vi "Convert Raw Bus Monitor Log.vi"(7 "48-bit Timetag?":bool, 8 "error in (no error)":errorcluster, 11 "Raw Bus Monitor Log":u16[](array[numeric])) -> (0 "error out":errorcluster, 3 "Formatted Bus Monitor Log":string[][](array[string]))   [LabVIEW 2016, in "BCI-1553 API.lvlib" / "1553 Component.lvclass"]
doc: "Converts a raw bus monitor log to a human-readable format. The first row is a header."
uses:
  1553 Component.lvclass
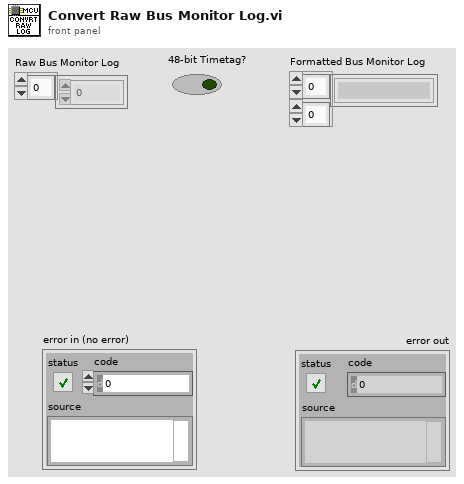
[diagram p1: front panel]
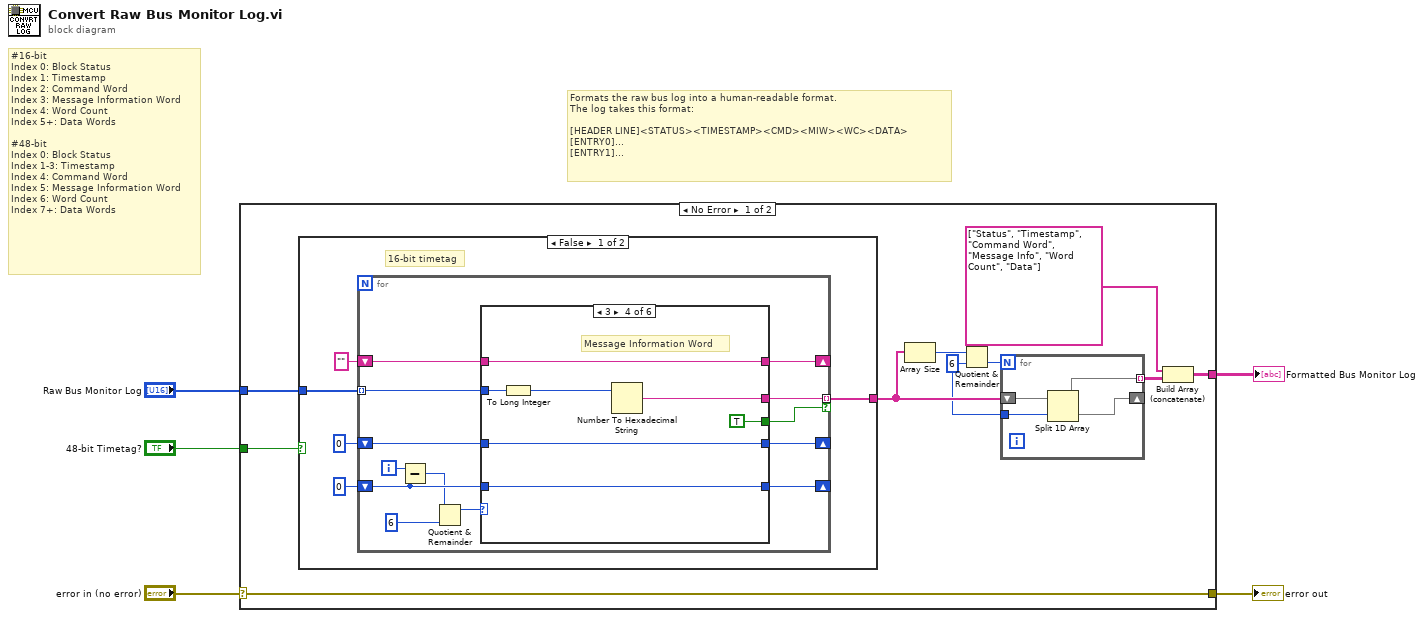
[diagram p0: block diagram]
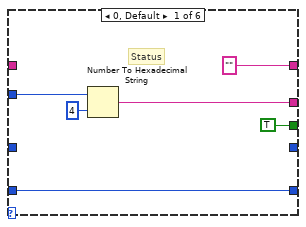
[diagram p2: hidden frame]
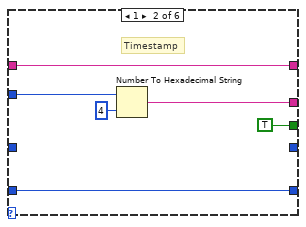
[diagram p3: hidden frame]
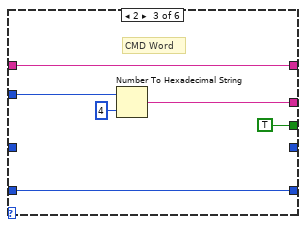
[diagram p4: hidden frame]
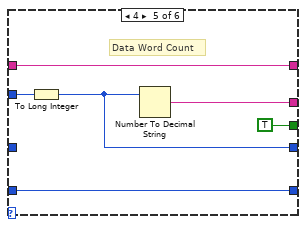
[diagram p5: hidden frame]
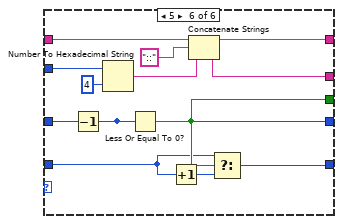
[diagram p6: hidden frame]
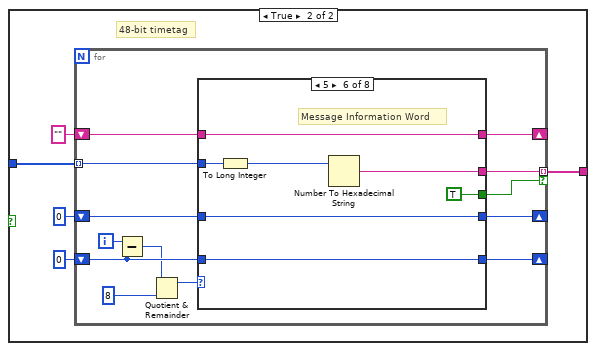
[diagram p7: hidden frame]
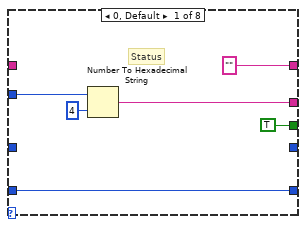
[diagram p8: hidden frame]
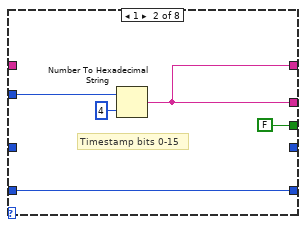
[diagram p9: hidden frame]
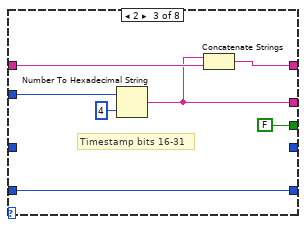
[diagram p10: hidden frame]
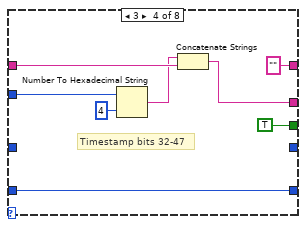
[diagram p11: hidden frame]
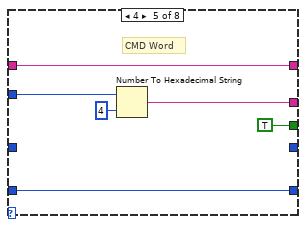
[diagram p12: hidden frame]
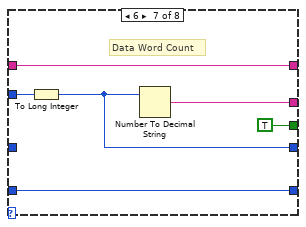
[diagram p13: hidden frame]
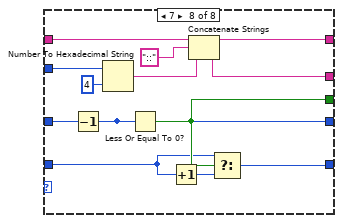
[diagram p14: hidden frame]
diagram:
  # "#16-bit\nIndex 0: Block Status\nIndex 1: Timestamp\nIndex 2: Command Word\nIndex 3: Message Information Word\nIndex 4: Word Count\nIndex 5+: Data Words\n\n#48-bit\nIndex 0: Block Status\nIndex 1-3: Timestamp\nIndex 4: Command Word\nIndex 5: Message Information Word\nIndex 6: Word Count\nIndex 7+: Data Words"
  # "Formats the raw bus log into a human-readable format.\nThe log takes this format:\n\n[HEADER LINE]<STATUS><TIMESTAMP><CMD><MIW><WC><DATA>\n[ENTRY0]...\n[ENTRY1]..."
  n1 = case shown="No Error" "error in (no error)" {
    selector: "error in (no error)" -> [w15 w156]
    tunnel: [w15 w156] -> w2
    tunnel: "Raw Bus Monitor Log" -> [w14 _]
    tunnel: [w8 _] -> w3
    tunnel: "48-bit Timetag?" -> [w6 _]
    frame No Error {
      w10 = 6 ("y")
      n2 = case shown="False" w6 {
        tunnel: w14 -> [w20 w78]
        tunnel: [w16 w77] -> w13
        frame False {
          # "16-bit timetag"
          n3 = for {
            tunnel: w20 -> [w27] mode=indexing
            shift-right: [w31] -> _
            shift-left: 0 ("y") -> [w29]
            tunnel: [w26] -> w16 mode=indexing if=w23
            shift-right: [w25] -> _
            shift-left: "" -> [w24]
            shift-right: [w22] -> _
            shift-left: 0 -> [w21]
            i -> [w30]
            n4 = Subtract(x=w30, y=w29) -> (x-y=w28:i32)
            n5 = Quotient & Remainder(x=w28, y=6) -> (x-y*floor(x/y)=w32:i32)  [unwired: 1 out]
            n6 = case shown="3" w32 {
              tunnel: w29 -> [w39 w45 w51 w54 w60 w70]
              tunnel: [w39 w45 w51 w54 w60 w68] -> w31
              tunnel: w27 -> [w38 w42 w48 w56 w62 w76]
              tunnel: [w36 w41 w47 w55 w61 w72] -> w26
              tunnel: ["" w44 w50 w58 w64 w72] -> w25
              tunnel: w24 -> [_ w44 w50 w58 w64 w66]
              tunnel: [TRUE TRUE TRUE TRUE TRUE w71] -> w23
              tunnel: [_ _ _ w52 w59 w67] -> w22
              tunnel: w21 -> [_ _ _ w52 _ w74]
              frame 0, Default {
                # "Status"
                n7 = Number To Hexadecimal String(1:i16 4 ("width (-)"), 2:w38) -> (0:w36:string)
              }
              frame 1 {
                # "Timestamp"
                n8 = Number To Hexadecimal String(1:i16 4 ("width (-)"), 2:w42) -> (0:w41:string)
              }
              frame 2 {
                # "CMD Word"
                n9 = Number To Hexadecimal String(1:i16 4 ("width (-)"), 2:w48) -> (0:w47:string)
              }
              frame 3 {
                # "Message Information Word"
                n10 = To Long Integer(number=w56) -> (32bit integer=w53:i32)
                n11 = Number To Hexadecimal String(2:w53) -> (0:w55:string)  [unwired: 1 in]
              }
              frame 4 {
                # "Data Word Count"
                n12 = To Long Integer(number=w62) -> (32bit integer=w59:i32)
                n13 = Number To Decimal String(number=w59) -> (decimal integer string=w61:string)  [unwired: 1 in]
              }
              frame 5 {
                n14 = Decrement(x=w74) -> (x-1=w67:i32)
                n15 = Number To Hexadecimal String(1:i16 4 ("width (-)"), 2:w76) -> (0:w65:string)
                n16 = Less Or Equal To 0?(x=w67) -> (x <= 0?=w71:bool)
                n17 = Increment(x=w70) -> (x+1=w69:i32)
                n18 = Concatenate Strings(w66, "::" ("string"), w65) -> (w72:string)
                n19 = Select(t=w70, s=w71, f=w69) -> (s? t:f=w68:i32)
              }
            }
          }
        }
        frame True {
          # "48-bit timetag"
          n20 = for {
            tunnel: w78 -> [w88] mode=indexing
            shift-right: [w92] -> _
            shift-left: 0 ("y") -> [w90]
            tunnel: [w87] -> w77 mode=indexing if=w84
            shift-right: [w86] -> _
            shift-left: "" -> [w85]
            shift-right: [w83] -> _
            shift-left: 0 -> [w82]
            i -> [w91]
            n21 = Subtract(x=w91, y=w90) -> (x-y=w89:i32)
            n22 = Quotient & Remainder(x=w89, y=8) -> (x-y*floor(x/y)=w93:i32)  [unwired: 1 out]
            n23 = case shown="5" w93 {
              tunnel: w90 -> [w100 w105 w112 w120 w126 w129 w135 w145]
              tunnel: [w100 w105 w112 w120 w126 w129 w135 w143] -> w92
              tunnel: w88 -> [w99 w103 w110 w118 w123 w131 w137 w151]
              tunnel: [w97 w101 w107 w113 w122 w130 w136 w147] -> w87
              tunnel: ["" w101 w106 "" w125 w133 w139 w147] -> w86
              tunnel: w85 -> [_ _ w108 w115 w125 w133 w139 w141]
              tunnel: [TRUE FALSE FALSE TRUE TRUE TRUE TRUE w146] -> w84
              tunnel: [_ _ _ _ _ w127 w134 w142] -> w83
              tunnel: w82 -> [_ _ _ _ _ w127 _ w149]
              frame 0, Default {
                # "Status"
                n24 = Number To Hexadecimal String(1:i16 4 ("width (-)"), 2:w99) -> (0:w97:string)
              }
              frame 1 {
                # "Timestamp bits 0-15"
                n25 = Number To Hexadecimal String(1:i16 4 ("width (-)"), 2:w103) -> (0:w101:string)
              }
              frame 2 {
                # "Timestamp bits 16-31"
                n26 = Number To Hexadecimal String(1:i16 4 ("width (-)"), 2:w110) -> (0:w107:string)
                n27 = Concatenate Strings(w107, w108) -> (w106:string)
              }
              frame 3 {
                # "Timestamp bits 32-47"
                n28 = Number To Hexadecimal String(1:i16 4 ("width (-)"), 2:w118) -> (0:w114:string)
                n29 = Concatenate Strings(w114, w115) -> (w113:string)
              }
              frame 4 {
                # "CMD Word"
                n30 = Number To Hexadecimal String(1:i16 4 ("width (-)"), 2:w123) -> (0:w122:string)
              }
              frame 5 {
                # "Message Information Word"
                n31 = To Long Integer(number=w131) -> (32bit integer=w128:i32)
                n32 = Number To Hexadecimal String(2:w128) -> (0:w130:string)  [unwired: 1 in]
              }
              frame 6 {
                # "Data Word Count"
                n33 = To Long Integer(number=w137) -> (32bit integer=w134:i32)
                n34 = Number To Decimal String(number=w134) -> (decimal integer string=w136:string)  [unwired: 1 in]
              }
              frame 7 {
                n35 = Decrement(x=w149) -> (x-1=w142:i32)
                n36 = Number To Hexadecimal String(1:i16 4 ("width (-)"), 2:w151) -> (0:w140:string)
                n37 = Less Or Equal To 0?(x=w142) -> (x <= 0?=w146:bool)
                n38 = Increment(x=w145) -> (x+1=w144:i32)
                n39 = Concatenate Strings(w141, "::" ("string"), w140) -> (w147:string)
                n40 = Select(t=w145, s=w146, f=w144) -> (s? t:f=w143:i32)
              }
            }
          }
        }
      }
      n41 = Array Size(array=w13) -> (size(s)=w12:i32)
      n42 = Quotient & Remainder(x=w12, y=w10) -> (floor(x/y)=w11:i32)  [unwired: 1 out]
      n43 = for {
        N: w11 -> [_]
        tunnel: w10 -> [w152]
        shift-right: [w154] -> _
        shift-left: w13 -> [w155]
        tunnel: [w153] -> w9 mode=indexing
        n44 = Split 1D Array(array=w155, index=w152) -> (first subarray=w153:string[], second subarray=w154:string[])
      }
      n45 = Build Array (concatenate)(string[] ["Status", "Timestamp", "Command Word", "Message Info", "Word Count", "Data"], w9) -> (w8:string[][])
    }
    frame Error {
    }
  }
  "error out" <- w2
  "Formatted Bus Monitor Log" <- w3
